vi "Scale Values.vi"(11 "Value":dbl) -> (3 "Value scaled":dbl)   [LabVIEW 2011]
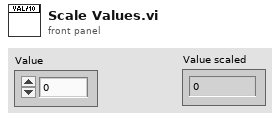
[diagram p1: front panel]
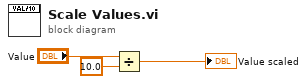
[diagram p0: block diagram]
diagram:
  n1 = Divide(x="Value", y=10.0) -> (x/y=→"Value scaled":dbl)
